vi "setNumberOfWheels.vi"(8 "error in (no error)":errorcluster, 10 "numberOfWheels":dbl, 11 "vehicleGeneric in":refnum<class "vehicleGeneric.lvclass">) -> (0 "error out":errorcluster, 3 "vehicleGeneric out":refnum<class "vehicleGeneric.lvclass">)   [LabVIEW 2011, in "vehicleGeneric.lvclass"]
uses:
  vehicleGeneric.lvclass
  vehicleGeneric.lvclass/vehicleGeneric.ctl
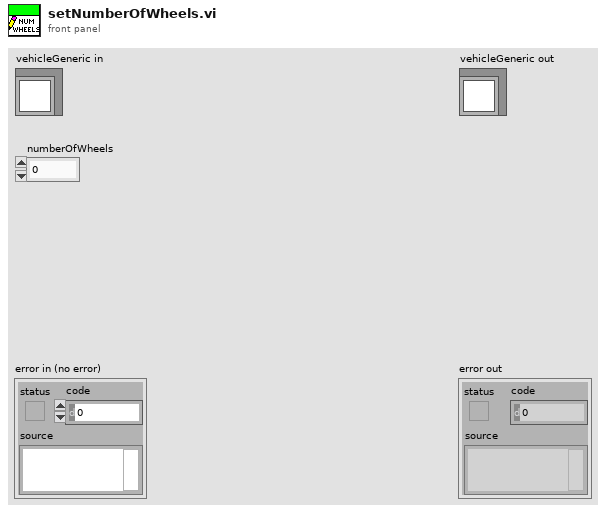
[diagram p1: front panel]
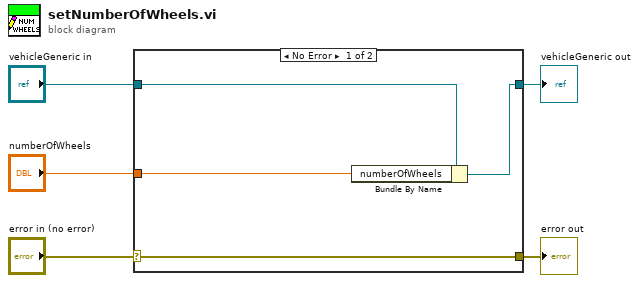
[diagram p0: block diagram]
diagram:
  n1 = case shown="No Error" "error in (no error)" {
    selector: "error in (no error)" -> [w9 w10]
    tunnel: [w9 w10] -> w4
    tunnel: [w7 w11] -> w2
    tunnel: "vehicleGeneric in" -> [w8 w11]
    tunnel: "numberOfWheels" -> [w6 _]
    frame No Error {
      n2 = Bundle By Name(cluster=w8, "numberOfWheels"=w6) -> (w7:refnum<class "vehicleGeneric.lvclass">)
    }
    frame Error {
    }
  }
  "error out" <- w4
  "vehicleGeneric out" <- w2
